vi "creat Input Task.vi"(8 "error in":errorcluster caption="错误输入", 10 "Configuration":T5, 11 "taskArr in":refnum<k21>[](array[refnum])) -> (0 "error out":errorcluster caption="错误输出", 3 "taskArr out":refnum<k21>[](array[refnum]))   [LabVIEW 2016]
uses:
  Control/Configuration.ctl
  Control/TaskConfig.ctl
  Control/ChanConfig.ctl
  Control/ClockConfig.ctl
  <vilib>/DAQmx/create/channels.llb/DAQmx Create Channel (AI-Voltage-Basic).vi
  <vilib>/DAQmx/configure/timing.llb/DAQmx Timing (Sample Clock).vi
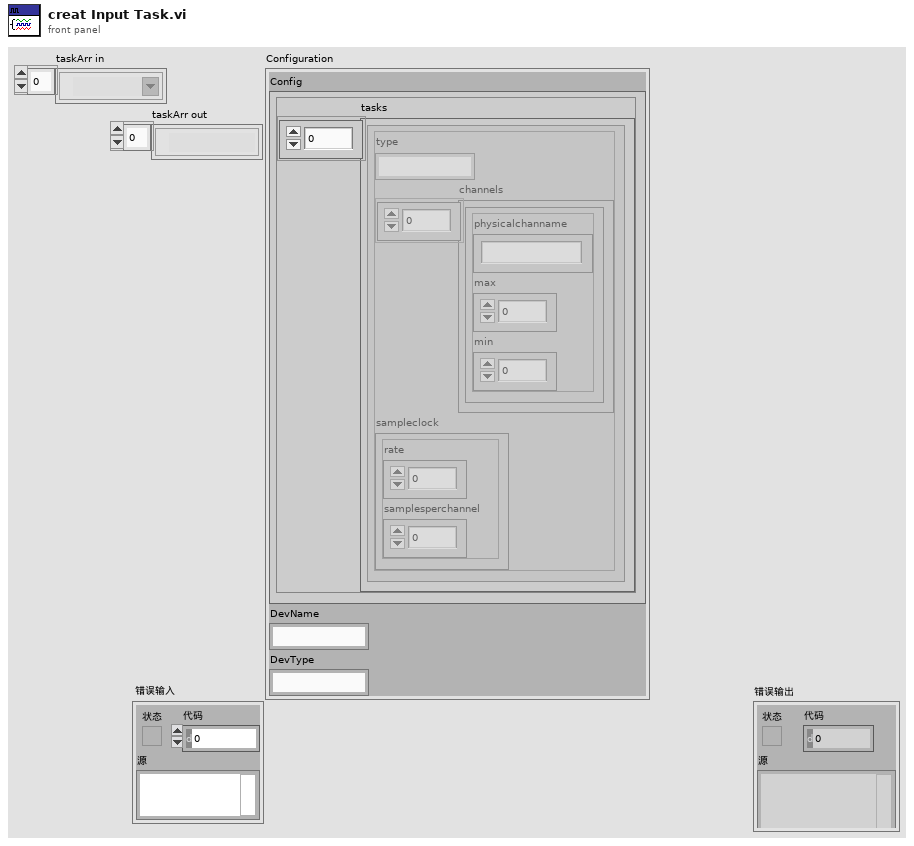
[diagram p1: front panel]
types:
  T1 = typedef "Configuration.ctl" = cluster{"tasks":T2[]}
  T2 = typedef "TaskConfig.ctl" = cluster{"type":string, "channels":T3[], "sampleclock":T4}
  T3 = typedef "ChanConfig.ctl" = cluster{"physicalchanname":string, "max":dbl, "min":dbl}
  T4 = typedef "ClockConfig.ctl" = cluster{"rate":dbl, "samplesperchannel":i32}
  T5 = cluster{"Config":T1, "DevName":string, "DevType":string}
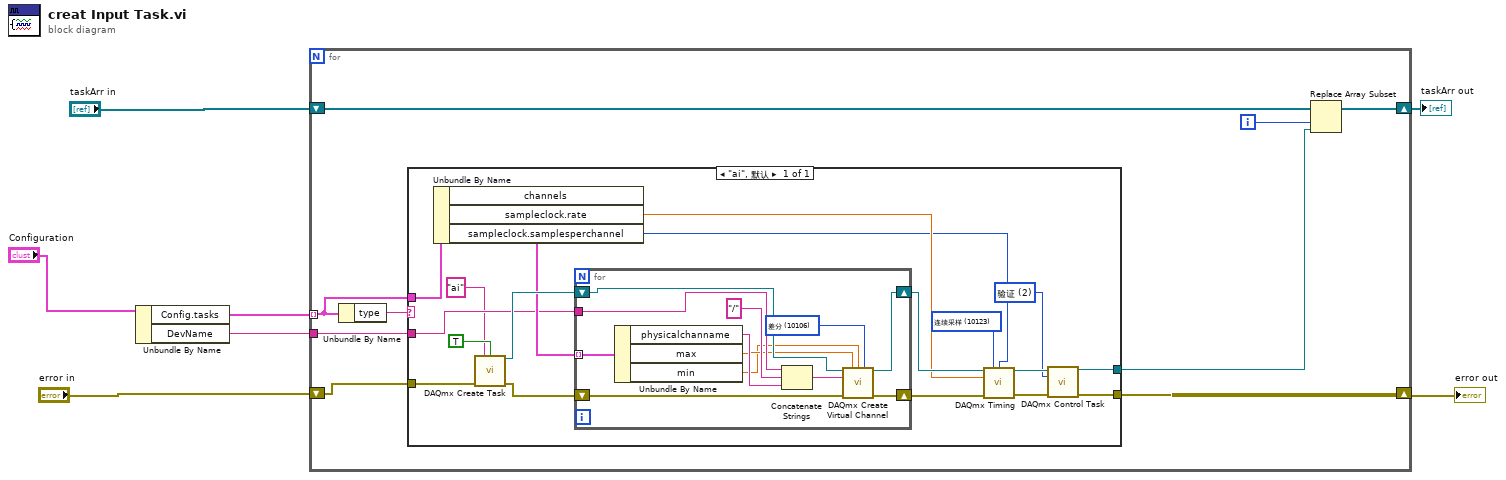
[diagram p0: block diagram]
diagram:
  n1 = Unbundle By Name("Configuration") -> ("Config.tasks"=w7:T2[], "DevName"=w6:string)
  n2 = for {
    tunnel: w7 -> [w15] mode=indexing
    tunnel: w6 -> [w14]
    shift-right: [w12] -> w4
    shift-left: "error in" -> [w13]
    shift-right: [w10] -> w2
    shift-left: "taskArr in" -> [w11]
    i -> [w9]
    n3 = Unbundle By Name(w15) -> ("type"=w16:string)
    n4 = case shown="\"ai\", 默认" w16 {
      tunnel: w15 -> [w32]
      tunnel: w14 -> [w30]
      tunnel: [w20] -> w12
      tunnel: w13 -> [w19]
      tunnel: [w18] -> w8
      frame "ai", Default {
        w22 = 2 items=["验证"=2, "保留"=4, "提交"=3, "未保留"=5, "中止"=6] ("action")
        w28 = 10123 items=["有限采样"=10178, "连续采样"=10123, "硬件定时单点"=12522] ("sample mode")
        n5 = Unbundle By Name(w32) -> ("channels"=w31:T3[], "sampleclock.rate"=w26:dbl, "sampleclock.samplesperchannel"=w25:i32)
        n6 = call <vilib>:"DAQmx Create Task.vi"("new task name"="ai", "auto cleanup"=TRUE, "error in"=w19) -> ("task out"=w33:refnum<k21>, "error out"=w21:errorcluster)  [unwired: 11 in]
        n7 = for {
          shift-right: [w43] -> w27
          shift-left: w33 -> [w44]
          shift-right: [w40] -> w29
          shift-left: w21 -> [w41]
          tunnel: w31 -> [w39] mode=indexing
          tunnel: w30 -> [w37]
          w42 = 10106 items=["默认"=-1, "RSE"=10083, "NRSE"=10078, "差分"=10106, "伪差分"=12529] ("input terminal configuration")
          n8 = Unbundle By Name(w39) -> ("physicalchanname"=w38:string, "max"=w36:dbl, "min"=w35:dbl)
          n9 = Concatenate Strings(w37, "/" ("字符串"), w38) -> (w45:string)
          n10 = call-poly <vilib>:"DAQmx Create Virtual Channel.vi"("task in"=w44, "maximum value"=w36, "minimum value"=w35, "input terminal configuration"=w42, "physical channels"=w45, "error in"=w41) -> ("task out"=w43:refnum<k21>, "error out"=w40:errorcluster)  [unwired: 8 in]
        }
        n11 = call-poly <vilib>:"DAQmx Timing.vi"("task/channels in"=w27, "sample mode"=w28, "samples per channel"=w25, "rate"=w26, "error in"=w29) -> ("task out"=w24:refnum<k21>, "error out"=w23:errorcluster)  [unwired: 9 in]
        n12 = call <vilib>:"DAQmx Control Task.vi"("task/channels in"=w24, "action"=w22, "error in"=w23) -> ("task out"=w18:refnum<k21>, "error out"=w20:errorcluster)  [unwired: 11 in]
      }
    }
    n13 = Replace Array Subset(array=w11, new element=w8, index=w9) -> (w10:refnum<k21>[])
  }
  "error out" <- w4
  "taskArr out" <- w2
